vi "p1.vi"() -> ()   [LabVIEW 2021, in "d11.lvlib"]
uses:
  d11.lvlib
  23ab682c-6edb-4c2f-b720-a3211d4e771f.vi
  <vilib>/Comparison/Less/Less Functor/Less Functor.lvclass
  AOC/AOC.lvlib
  <vilib>/gmath/NI_Gmath.lvlib
panel:
  out "Monkeys":T1(array[cluster])=[{"ID."=0, "Items"=[3, 3, 3, 3, 4, 4, 4, 4, 4, 4, 4, 4, 1, 1, 1, 1, 1], "Operation"="y = x * 5", "Test"=3, "True"=7, "False"=4, "Count"=259}, {"ID."=1, "Items"=[3, 3, 3, 3, 6, 6], "Operation"="y = x + 6", "Test"=17, "True"=3, "False"=0, "Count"=140}, {"ID."=2, "Items"=[4, 4, 1, 1, 1, 1, 1, 1, 1, 1, 1, 1], "Operation"="y = x + 5", "Test"=2, "True"=3, "False"=1, "Count"=211}, {"ID."=3, "Items"=[], "Operation"="y = x + 2", "Test"=19, "True"=7, "False"=0, "Count"=133}, {"ID."=4, "Items"=[], "Operation"="y = x * 7", "Test"=11, "True"=5, "False"=6, "Count"=188}, {"ID."=5, "Items"=[], "Operation"="y = x + 7", "Test"=5, "True"=2, "False"=1, "Count"=66}, {"ID."=6, "Items"=[12], "Operation"="y = x + 1", "Test"=13, "True"=5, "False"=2, "Count"=216}, {"ID."=7, "Items"=[], "Operation"="y = x * x", "Test"=7, "True"=4, "False"=6, "Count"=83}]
  in  "Example":string="Monkey 0:\n  Starting items: 79, 98\n  Operation: new = old * 19\n  Test: divisible by 23\n    If true: throw to monkey 2\n    If false: throw to monkey 3\n\nMonkey 1:\n  Starting items: 54, 65, 75, 74\n  Operation: new = old + 6\n  Test: divisible by 19\n    If true: throw to monkey 2\n    If false: throw to monkey 0\n\nMonkey 2:\n  Starting items: 79, 60, 97\n  Operation: new = old * old\n  Test: divisible by 13\n    If true: throw to monkey 1\n    If false: throw to monkey 3\n\nMonkey 3:\n  Starting items: 74\n  Operation: new = old + 3\n  Test: divisible by 17\n    If true: throw to monkey 0\n    If false: throw to monkey 1"
  in  "Example":bool
  out "Answer":i64=55944
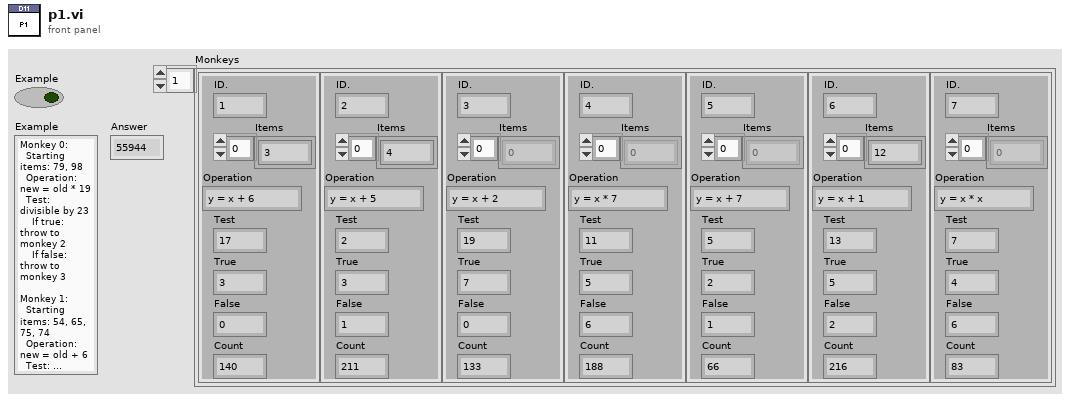
[diagram p1: front panel]
types:
  T1 = cluster{"ID.":i64, "Items":i64[], "Operation":string, "Test":i64, "True":i64, "False":i64, "Count":i64}[]
  T2 = cluster{"ID.":i64, "Items":i64[], "Operation":string, "Test":i64, "True":i64, "False":i64, "Count":i64}
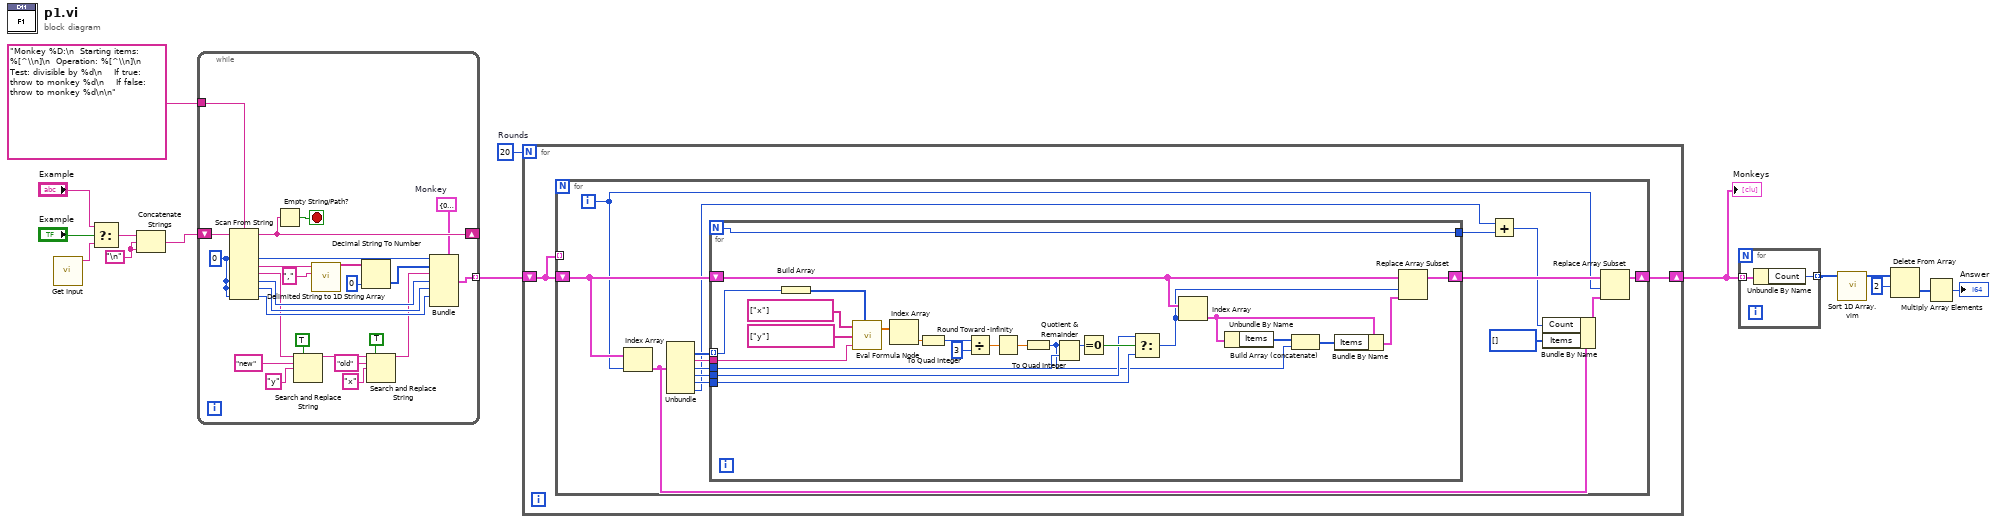
[diagram p0: block diagram]
diagram:
  w7 = "\n"
  w9 = 20  # Rounds
  n1 = call "Get Input.vi"() -> ("Input"=w15:string)  [unwired: 11 in]
  n2 = Select(t="Example", s="Example", f=w15) -> (s? t:f=w12:string)
  n3 = Concatenate Strings(w12, w7, w7) -> (w8:string)
  n4 = while {
    shift-right: [w37] -> _
    shift-left: w8 -> [w40]
    tunnel: "Monkey %D:\n  Starting items: %[^\\n]\n  Operation: %[^\\n]\n  Test: divisible by %d\n    If true: throw to monkey %d\n    If false: throw to monkey %d\n\n" ("format string") -> [w39]
    tunnel: [w29] -> w10 mode=indexing
    stop <- w38 stop-if-true
    w26 = i64 0 ("default value 1")
    w27 = T2 {"ID."=0, "Items"=[], "Operation"="", "Test"=0, "True"=0, "False"=0, "Count"=0}  # Monkey
    n5 = Scan From String(format string=w39, input string=w40, default 1=w26, default 4=w26, default 5=w26, default 6=w26) -> (remaining string=w37:string, output 1=w34:i64, output 2=w35:string, output 3=w24:string, output 4=w32:i64, output 5=w31:i64, output 6=w30:i64)  [unwired: 4 in, 2 out]
    n6 = Empty String/Path?(string/path=w37) -> (empty?=w38:bool)
    n7 = Search and Replace String(replace all?=TRUE ("replace all? (F)"), input string=w24, search string="new" ("input string"), replace string="y" ("replace string (\"\")")) -> (result string=w20:string)  [unwired: 4 in, 3 out]
    n8 = call <vilib>:"Delimited String to 1D String Array.vi"("delimiter"=",", "delimited string"=w35) -> ("string array"=w33:string[])  [unwired: 9 in]
    n9 = Decimal String To Number(string=w33, default (0L)=i64 0 ("default (0 I32)")) -> (number=w28:i64[])  [unwired: 1 in, 1 out]
    n10 = Search and Replace String(replace all?=TRUE ("replace all? (F)"), input string=w20, search string="old", replace string="x" ("replace string (\"\")")) -> (result string=w21:string)  [unwired: 4 in, 3 out]
    n11 = Bundle(cluster=w27, "ID."=w34, "Items"=w28, "Operation"=w21, "Test"=w32, "True"=w31, "False"=w30) -> (w29:T2)  [unwired: 1 in]
  }
  n12 = for {
    N: w9 -> [_]
    shift-right: [w41] -> w6
    shift-left: w10 -> [w42]
    n13 = for {
      shift-right: [w49] -> w41
      shift-left: w42 -> [w52]
      tunnel: w42 -> [_] mode=indexing
      i -> [w47]
      n14 = Index Array(array=w52, index=w47) -> (element=w46:T2)
      n15 = Unbundle(w46) -> ("Items"=w56:i64[], "Operation"=w57:string, "Test"=w55:i64, "True"=w54:i64, "False"=w53:i64, "Count"=w44:i64)  [unwired: 1 out]
      n16 = for {
        N -> [w58]
        tunnel: w57 -> [w80]
        tunnel: w56 -> [w79] mode=indexing
        tunnel: w55 -> [w76]
        tunnel: w54 -> [w73]
        tunnel: w53 -> [w72]
        shift-right: [w69] -> w50
        shift-left: w52 -> [w70]
        tunnel: [w58] -> w45
        n17 = Build Array(w79) -> (w78:i64[])
        n18 = call <vilib>:"Eval Formula Node.vi"("Variables Input"=string[] ["x"], "Input Values"=w78, "Variables Output"=string[] ["y"], "formula"=w80) -> ("Output Values"=w77:dbl[])  [unwired: 1 in, 1 out]
        n19 = Index Array(array=w77) -> (element=w64:dbl)  [unwired: 1 in]
        n20 = To Quad Integer(1:w64) -> (0:w63:i64)
        n21 = Divide(x=w63, y=i64 3) -> (x/y=w62:dbl)
        n22 = Round Toward -Infinity(1:w62) -> (0:w60:dbl)
        n23 = To Quad Integer(1:w60) -> (0:w59:i64)
        n24 = Quotient & Remainder(x=w59, y=w76) -> (x-y*floor(x/y)=w75:i64)  [unwired: 1 out]
        n25 = Equal To 0?(x=w75) -> (x = 0?=w74:bool)
        n26 = Select(t=w73, s=w74, f=w72) -> (s? t:f=w68:i64)
        n27 = Index Array(array=w70, index=w68) -> (element=w67:T2)
        n28 = Unbundle By Name(w67) -> ("Items"=w71:i64[])
        n29 = Build Array (concatenate)(w71, w59) -> (w66:i64[])
        n30 = Bundle By Name(cluster=w67, "Items"=w66) -> (w65:T2)
        n31 = Replace Array Subset(array=w70, new element=w65, index=w68) -> (w69:T1)
      }
      n32 = Add(x=w44, y=w45) -> (x+y=w43:i64)
      n33 = Bundle By Name(cluster=w46, "Count"=w43, "Items"=i64[] []) -> (w48:T2)
      n34 = Replace Array Subset(array=w50, new element=w48, index=w47) -> (w49:T1)
    }
  }
  "Monkeys" <- w6
  n35 = for {
    tunnel: w6 -> [w84] mode=indexing
    tunnel: [w83] -> w5 mode=indexing
    n36 = Unbundle By Name(w84) -> ("Count"=w83:i64)
  }
  n37 = call "Sort 1D Array.vim"("unsorted array"=w5) -> ("sorted array"=w4:i64[])  [unwired: 10 in]
  n38 = Delete From Array(array=w4, length=2) -> (deleted portion=w1:i64[])  [unwired: 1 in, 1 out]
  n39 = Multiply Array Elements(1:w1) -> (0:→"Answer":i64)
